vi "TestAllReadings.vi"() -> ()   [LabVIEW 2017]
uses:
  InputRange.ctl
  InputType.ctl
  InputMode.ctl
  DataChannel.ctl
  DataFrontPanel.ctl
  InputCouple.ctl
  InputFilter.ctl
  InputGround.ctl
  InputSensitivity.ctl
  InputTimeConstant.ctl
  OutputChannelSignal.ctl
  OutputChannel.ctl
  OutSineReference.ctl
  OutSineSource.ctl
panel:
  out "error out":errorcluster
  out "OutSineSource":T1 caption="Out sine ref" items=["Internal", "External", "Dual", "Chop"]
  out "OutSineRef":T2 caption="Out sine ref" items=["Common", "Difference"]
  out "Offset":dbl caption="Offset, V"
  out "Frequency":dbl caption="Frequency, Hz"
  out "Amplitude":dbl caption="Amplitude, V"
  in  "OutputChannel":T3 caption="Output channel" items=["Channel 1", "Channel 2"]
  out "OutputChannelSignal":T4 caption="Output channel signal" items=["X (ch1) / Y (ch2)", "R (ch1) / Q (ch2)"]
  out "InputTimeConstant":T5=2 caption="Input time constant" items=["1 us", "3 us", "10 us", "30 us", "100 us", "300 us", "1 ms", "3 ms", "10 ms", "30 ms", "100 ms", "300 ms", "1 s", "3 s", "10 s", "30 s", "100 s", "300 s", "1 Ks", "3 Ks", "10 Ks", "30 Ks"]
  out "InputSensitivity":T6=26 caption="Input sensitivity" items=["1 V [uA]", "500 mV [nA]", "200 mV [nA]", "100 mV [nA]", "50 mV [nA]", "20 mV [nA]", "10 mV [nA]", "5 mV [nA]", "2 mV [nA]", "1 mV [nA]", "500 uV [pA]", "200 uV [pA]", "100 uV [pA]", "50 uV [pA]", "20 uV [pA]", "10 uV [pA]", "5 uV [pA]", "2 uV [pA]", "1 uV [pA]", "500 nV [fA]", "200 nV [fA]", "100 nV [fA]", "50 nV [fA]", "20 nV [fA]", "10 nV [fA]", "5 nV [fA]", "2 nV [fA]", "1 nV [fA]"]
  out "InputGround":T7 caption="Input ground" items=["Float", "Ground"]
  out "InputFilter":T8 caption="Input filter" items=["6 db/oct", "12 db/oct", "18 db/oct", "24 db/oct"]
  out "InputCouple":T9 caption="Input couple" items=["AC", "DC"]
  out "Data 2":dbl caption="Data"
  in  "DataFrontPanel":T10=2 caption="Data channel" items=["Green", "Blue", "Yellow", "Orange"]
  out "Data":dbl
  in  "DataChannel":T11=2 caption="Data channel" items=["X", "Y", "R", "Theta", "IN1", "IN2", "IN3", "IN4", "OUT1", "OUT2", "XNoise", "YNoise", "Phase", "SineOut", "DCLevel", "IntRefFreq", "ExtRefFreq"]
  out "InputMode":T12 caption="Input mode" items=["A", "A-B"]
  out "InputType":T13=2 caption="Input type" items=["Voltage", "Current"]
  out "InputRange":T14=2 caption="Input range" items=["1 V", "300 mV", "100 mV", "30 mV", "10 mV"]
  in  "VISA resource name":refnum<visa-resource-name>
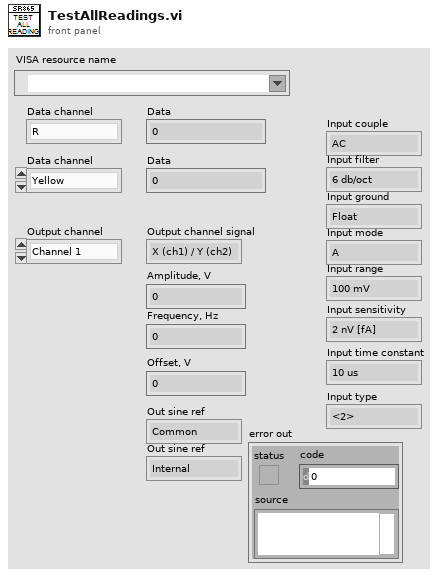
[diagram p1: front panel]
types:
  T1 = typedef "OutSineSource.ctl" = u16
  T2 = typedef "OutSineReference.ctl" = u16
  T3 = typedef "OutputChannel.ctl" = u16
  T4 = typedef "OutputChannelSignal.ctl" = u16
  T5 = typedef "InputTimeConstant.ctl" = u16
  T6 = typedef "InputSensitivity.ctl" = u16
  T7 = typedef "InputGround.ctl" = u16
  T8 = typedef "InputFilter.ctl" = u16
  T9 = typedef "InputCouple.ctl" = u16
  T10 = typedef "DataFrontPanel.ctl" = u16
  T11 = typedef "DataChannel.ctl" = u16
  T12 = typedef "InputMode.ctl" = u16
  T13 = typedef "InputType.ctl" = u16
  T14 = typedef "InputRange.ctl" = u16
  T15 = typedef "SR865.ctl" = cluster{"VISA resource name":refnum<visa-resource-name>, "ReadWrite":T16}
  T16 = typedef "Semaphore RefNum" = refnum<k1>
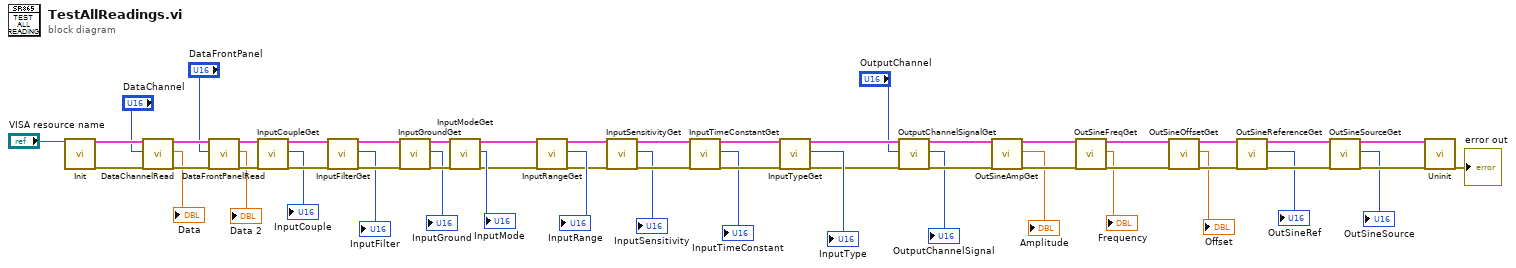
[diagram p0: block diagram]
diagram:
  n1 = call "Init.vi"("VISA resource name"="VISA resource name") -> ("SR865"=w51:T15, "error out"=w34:errorcluster)  [unwired: 17 in]
  n2 = call "DataChannelRead.vi"("SR865 in"=w51, "DataChannel"="DataChannel", "error in"=w34) -> ("SR865 out"=w50:T15, "Signal"=→"Data":dbl, "error out"=w33:errorcluster)  [unwired: 14 in]
  n3 = call "DataFrontPanelRead.vi"("SR865 in"=w50, "DataFrontPanel"="DataFrontPanel", "error in"=w33) -> ("SR865 out"=w49:T15, "Data"=→"Data 2":dbl, "error out"=w32:errorcluster)  [unwired: 14 in]
  n4 = call "InputCoupleGet.vi"("SR865 in"=w49, "error in"=w32) -> ("SR865 out"=w48:T15, "InputCouple"=→"InputCouple":T9, "error out"=w31:errorcluster)  [unwired: 15 in]
  n5 = call "InputFilterGet.vi"("SR865 in"=w48, "error in"=w31) -> ("SR865 out"=w47:T15, "InputFilter"=→"InputFilter":T8, "error out"=w30:errorcluster)  [unwired: 15 in]
  n6 = call "InputGroundGet.vi"("SR865 in"=w47, "error in"=w30) -> ("SR865 out"=w46:T15, "InputGround"=→"InputGround":T7, "error out"=w29:errorcluster)  [unwired: 15 in]
  n7 = call "InputModeGet.vi"("SR865 in"=w46, "error in"=w29) -> ("SR865 out"=w45:T15, "InputMode"=→"InputMode":T12, "error out"=w28:errorcluster)  [unwired: 15 in]
  n8 = call "InputRangeGet.vi"("SR865 in"=w45, "error in"=w28) -> ("SR865 out"=w44:T15, "InputRange"=→"InputRange":T14, "error out"=w27:errorcluster)  [unwired: 15 in]
  n9 = call "InputSensitivityGet.vi"("SR865 in"=w44, "error in"=w27) -> ("SR865 out"=w43:T15, "InputSensitivity"=→"InputSensitivity":T6, "error out"=w26:errorcluster)  [unwired: 15 in]
  n10 = call "InputTimeConstantGet.vi"("SR865 in"=w43, "error in"=w26) -> ("SR865 out"=w42:T15, "InputTimeConstant"=→"InputTimeConstant":T5, "error out"=w25:errorcluster)  [unwired: 15 in]
  n11 = call "InputTypeGet.vi"("SR865 in"=w42, "error in"=w25) -> ("SR865 out"=w41:T15, "InputType"=→"InputType":T13, "error out"=w24:errorcluster)  [unwired: 15 in]
  n12 = call "OutputChannelSignalGet.vi"("SR865 in"=w41, "OutputChannel"="OutputChannel", "error in"=w24) -> ("SR865 out"=w40:T15, "OutputChannelSignal"=→"OutputChannelSignal":T4, "error out"=w23:errorcluster)  [unwired: 14 in]
  n13 = call "OutSineAmpGet.vi"("SR865 in"=w40, "error in"=w23) -> ("SR865 out"=w39:T15, "Amplitude"=→"Amplitude":dbl, "error out"=w22:errorcluster)  [unwired: 15 in]
  n14 = call "OutSineFreqGet.vi"("SR865 in"=w39, "error in"=w22) -> ("SR865 out"=w38:T15, "Frequency"=→"Frequency":dbl, "error out"=w21:errorcluster)  [unwired: 15 in]
  n15 = call "OutSineOffsetGet.vi"("SR865 in"=w38, "error in"=w21) -> ("SR865 out"=w37:T15, "Offset"=→"Offset":dbl, "error out"=w20:errorcluster)  [unwired: 15 in]
  n16 = call "OutSineReferenceGet.vi"("SR865 in"=w37, "error in"=w20) -> ("SR865 out"=w36:T15, "OutSineRef"=→"OutSineRef":T2, "error out"=w19:errorcluster)  [unwired: 15 in]
  n17 = call "OutSineSourceGet.vi"("SR865 in"=w36, "error in"=w19) -> ("SR865 out"=w35:T15, "OutSineSource"=→"OutSineSource":T1, "error out"=w18:errorcluster)  [unwired: 15 in]
  n18 = call "Uninit.vi"("SR865 in"=w35, "error in"=w18) -> ("error out"=→"error out":errorcluster)  [unwired: 17 in]
